vi "Example.vi"(3 "Table Content":T1={"TableHeader"=["Soll\nppm/%", "Ist\nppm/%", "Fehler\n%", "Toleranz\n%", "Ergebnis"], "Table"=[["aaa", "bbb", "ccc", "ddd"], ["111", "222", "333", "444"], ["sss", "fff", "kkk", "xxx"], ["6.5", "11.13", "19.2", "4"], ["1111", "1212", "777", "888"]], "Relative Column Widths (%)"=[22.5, 22.5, 22.5, 22.5, 4.0], "Results"={"Results"=[], "ResultPictures"={"Yes Ctl Refnum"=refnum, "No Ctl Refnum"=refnum}, "use Pictures"=FALSE}, "PositionBemerkung"=enum."before", "PageBreak"=enum."before", "TablePictures"={"Ctl Refnum In"=[], "RowOrColumn"=enum."Row", "IndexToInsert"=0, "Image Scale (%)"=[], "Autoscale? (T)"=[], "Horizontal Align"=3}, "Horizontal Align"=3} {"Horizontal Align" items=["Center", "Justified", "JustifiedAll", "Left", "Right"]; "TablePictures"."Horizontal Align" items=["Center", "Justified", "JustifiedAll", "Left", "Right"]}) -> (11 "XY-Graph":cluster{"X":dbl, "Y":dbl}[](graph))   [LabVIEW 2020, in "PDF Interface.lvlib"]
uses:
  PDF Interface.lvlib
  <vilib>/Simplicity AI/SAI_PDF_API/Classes/Context/Controls/SAI_PDF_Text Align.ctl
  <vilib>/Simplicity AI/SAI_PDF_API/Classes/Context/Context.lvclass
  PDF Interface Helper/PDFContentType.ctl
  PDF Interface Helper/PDF Interface Helper.lvlib
  <vilib>/Simplicity AI/SAI_PDF_API/Classes/Context/Controls/SAI_PDF_PDF Details.ctl
  PDF Interface Helper/PDFTableContentType.ctl
  PDF Interface Helper/PDFPageBreak.ctl
  PDF Interface Helper/PDFCommentPosition.ctl
  PDF Interface Helper/PDFTablePictures.ctl
  PDF Interface Helper/PDFResultPictures.ctl
  PDF Interface Helper/PDFResults.ctl
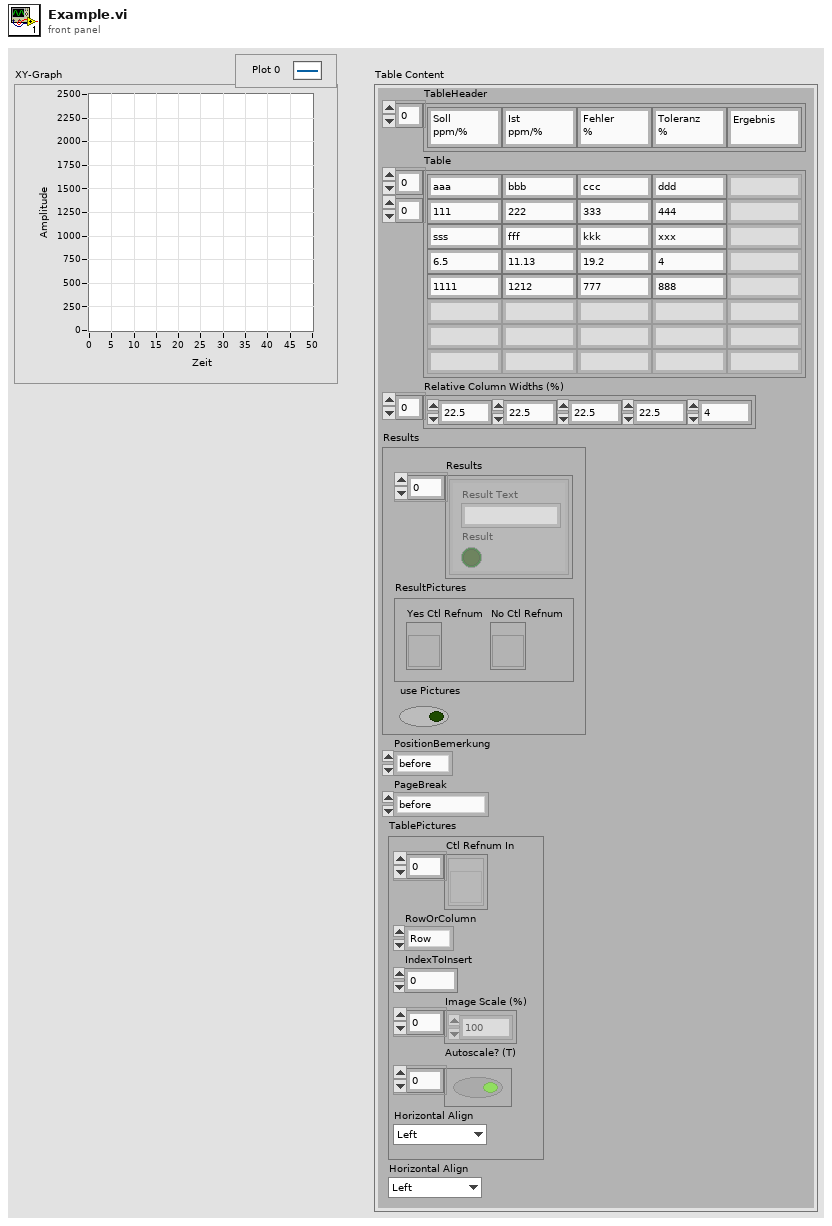
[diagram p1: front panel]
types:
  T1 = typedef "PDF Interface.lvlib/PDF Interface Helper.lvlib/PDFTableContentType.ctl" = cluster{"TableHeader":string[], "Table":string[][], "Relative Column Widths (%)":sgl[], "Results":T2, "PositionBemerkung":T4, "PageBreak":T5, "TablePictures":T6, "Horizontal Align":i32}
  T2 = typedef "PDF Interface.lvlib/PDF Interface Helper.lvlib/PDFResults.ctl" = cluster{"Results":cluster{"Result Text":string, "Result":bool}[], "ResultPictures":T3, "use Pictures":bool}
  T3 = typedef "PDF Interface.lvlib/PDF Interface Helper.lvlib/PDFResultPictures.ctl" = cluster{"Yes Ctl Refnum":refnum<vi>, "No Ctl Refnum":refnum<vi>}
  T4 = typedef "PDF Interface.lvlib/PDF Interface Helper.lvlib/PDFCommentPosition.ctl" = enum16{"before", "after"}
  T5 = typedef "PDF Interface.lvlib/PDF Interface Helper.lvlib/PDFPageBreak.ctl" = enum16{"none", "before", "after", "after comment"}
  T6 = typedef "PDF Interface.lvlib/PDF Interface Helper.lvlib/PDFTablePictures.ctl" = cluster{"Ctl Refnum In":refnum<vi>[], "RowOrColumn":enum16{"Row", "Column"}, "IndexToInsert":u16, "Image Scale (%)":sgl[], "Autoscale? (T)":bool[], "Horizontal Align":i32}
  T7 = typedef "PDF Interface.lvlib/PDF Interface Helper.lvlib/PDFContentType.ctl" = cluster{"Titel":string, "Header Table":string[][], "Table Array":T1[], "Bemerkungen":cluster{"Bemerkung Text":string, "Align (Left)":T8, "Add Line Feeds (F:No)":bool}[]}
  T8 = typedef "SAI_PDF_Toolkit.lvlib/Context.lvclass/SAI_PDF_Text Align.ctl" = i32
  T9 = cluster{"Bemerkung Text":string, "Align (Left)":T8, "Add Line Feeds (F:No)":bool}[]
  T10 = cluster{"GraphCtl Refnum":refnum<vi>, "Wrap Text (F:No)":bool, "Hide Grid (F:No)":bool, "Scale (100%)":sgl, "Align (Left)":T8}
  T11 = typedef "SAI_PDF_Toolkit.lvlib/Context.lvclass/SAI_PDF_PDF Details.ctl" = cluster{"Title":string, "Subject":string, "Keywords":string, "Author":string, "Creator":string}
  T12 = cluster{"Header Footer Text Cluster":cluster{"Header Text":string, "Footer Text":string, "Time":string, "Page Number":string}, "PDF Details":T11}
  T13 = cluster{"GraphCtl Refnum":refnum<vi>, "Wrap Text (F:No)":bool, "Hide Grid (F:No)":bool, "Scale (100%)":sgl, "Align (Left)":T8}[]
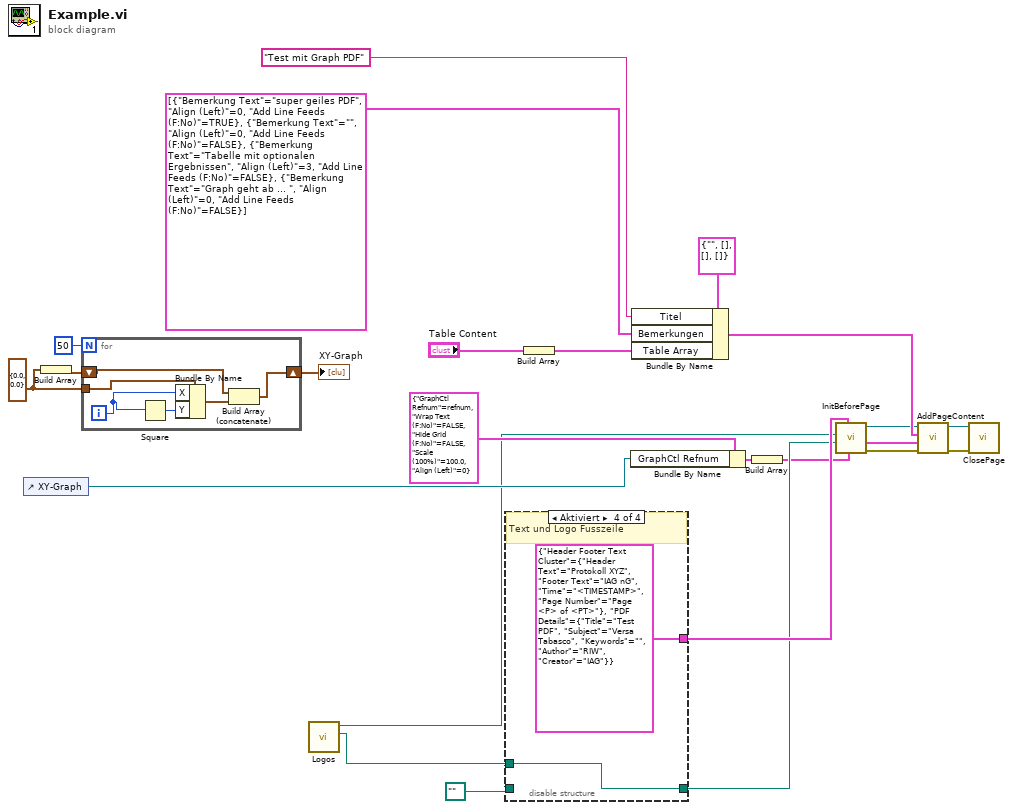
[diagram p0: block diagram]
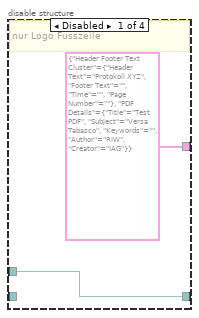
[diagram p2: hidden frame]
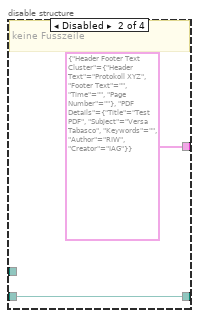
[diagram p3: hidden frame]
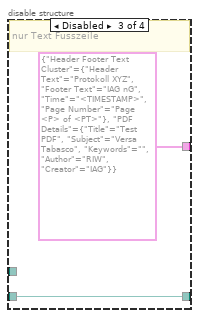
[diagram p4: hidden frame]
diagram:
  w20 = cluster{"X":dbl, "Y":dbl} {"X"=0.0, "Y"=0.0} ("XY-Graph")
  n1 = control-ref of="XY-Graph"() -> (w17:refnum<vi>)
  n2 = Build Array(w20) -> (w21:cluster{"X":dbl, "Y":dbl}[])
  n3 = for {
    N: 50 -> [_]
    shift-right: [w24] -> w22
    shift-left: w21 -> [w26]
    tunnel: w20 -> [w25]
    i -> [w28]
    n4 = Square(x=w28) -> (x^2=w29:i32)
    n5 = Bundle By Name(cluster=w25, "X"=w28, "Y"=w29) -> (w27:cluster{"X":dbl, "Y":dbl})
    n6 = Build Array (concatenate)(w26, w27) -> (w24:cluster{"X":dbl, "Y":dbl}[])
  }
  "XY-Graph" <- w22
  n7 = call "Logos.vi"() -> ("Footer Image File Path"=w12:path, "Header Image File Path"=w10:path)  [unwired: 9 in, 1 out]
  n8 = disable-structure shown="Aktiviert" {
    disable-tunnel: [T12 {"Header Footer Text Cluster"={"Header Text"="Protokoll XYZ", "Footer Text"="", "Time"="", "Page Number"=""}, "PDF Details"={"Title"="Test PDF", "Subject"="Versa Tabasco", "Keywords"="", "Author"="RIW", "Creator"="IAG"}} ("Info") T12 {"Header Footer Text Cluster"={"Header Text"="Protokoll XYZ", "Footer Text"="", "Time"="", "Page Number"=""}, "PDF Details"={"Title"="Test PDF", "Subject"="Versa Tabasco", "Keywords"="", "Author"="RIW", "Creator"="IAG"}} ("Info") T12 {"Header Footer Text Cluster"={"Header Text"="Protokoll XYZ", "Footer Text"="IAG nG", "Time"="<TIMESTAMP>", "Page Number"="Page <P> of <PT>"}, "PDF Details"={"Title"="Test PDF", "Subject"="Versa Tabasco", "Keywords"="", "Author"="RIW", "Creator"="IAG"}} ("Info") T12 {"Header Footer Text Cluster"={"Header Text"="Protokoll XYZ", "Footer Text"="IAG nG", "Time"="<TIMESTAMP>", "Page Number"="Page <P> of <PT>"}, "PDF Details"={"Title"="Test PDF", "Subject"="Versa Tabasco", "Keywords"="", "Author"="RIW", "Creator"="IAG"}} ("Info")] -> w11
    disable-tunnel: w12 -> [w30 _ _ w36]
    disable-tunnel: path "" ("Footer Image File Path") -> [_ w32 w34 _]
    disable-tunnel: [w30 w32 w34 w36] -> w9
    frame Disabled {
      # "nur Logo Fusszeile"
    }
    frame Disabled {
      # "keine Fusszeile"
    }
    frame Disabled {
      # "nur Text Fusszeile"
    }
    frame Enabled {
      # "Text und Logo Fusszeile"
    }
  }
  n9 = Build Array("Table Content") -> (w2:T1[])
  n10 = Bundle By Name(cluster=T10 {"GraphCtl Refnum"=refnum, "Wrap Text (F:No)"=FALSE, "Hide Grid (F:No)"=FALSE, "Scale (100%)"=100.0, "Align (Left)"=0} ("Graph"), "GraphCtl Refnum"=w17) -> (w18:T10)
  n11 = Bundle By Name(cluster=T7 {"Titel"="", "Header Table"=[], "Table Array"=[], "Bemerkungen"=[]} ("Content"), "Titel"="Test mit Graph PDF", "Bemerkungen"=T9 [{"Bemerkung Text"="super geiles PDF", "Align (Left)"=0, "Add Line Feeds (F:No)"=TRUE}, {"Bemerkung Text"="", "Align (Left)"=0, "Add Line Feeds (F:No)"=FALSE}, {"Bemerkung Text"="Tabelle mit optionalen Ergebnissen", "Align (Left)"=3, "Add Line Feeds (F:No)"=FALSE}, {"Bemerkung Text"="Graph geht ab ... ", "Align (Left)"=0, "Add Line Feeds (F:No)"=FALSE}], "Table Array"=w2) -> (w7:T7)
  n12 = Build Array(w18) -> (w3:T13)
  n13 = call "InitBeforePage.vi"("Info"=w11, "Footer Image File Path"=w9, "Header Image File Path"=w10) -> ("Fehler (Ausgang)"=w5:errorcluster, "Context (Ausgang)"=w4:refnum<class "Context.lvclass">)  [unwired: 7 in]
  n14 = call "AddPageContent.vi"("error in"=w5, "Graph Array"=w3, "Content"=w7, "Context (Eingang)"=w4) -> ("error out"=w8:errorcluster, "Context (Ausgang)"=w6:refnum<class "Context.lvclass">)  [unwired: 6 in]
  n15 = call "ClosePage.vi"("Fehler (Eingang, kein Fehler)"=w8, "Context (Eingang)"=w6) -> ()  [unwired: 9 in, 1 out]
